vi "XYStage.KIM101.GetProtectedEvents.vi"(8 "error in (no error)":errorcluster, 11 "XYStage.KIM101":refnum<class "XYStage.KIM101.lvclass">) -> (0 "error out":errorcluster, 2 "Protected Events":T1, 3 "XYStage.KIM101 out":refnum<class "XYStage.KIM101.lvclass">)   [LabVIEW 2017, in "XYStage.KIM101.lvclass"]
doc: "---------------------------------------------------------------\nJKI State Machine Objects™\nhttp://jki.net/state-machine-objects/\nCopyright (C) 2005-2015, JKI <info@jki.net>\nALL RIGHTS RESERVEDJKI State Machine Objects (SMO) 1.0.0.5\nJKI - JKI\nCopyright (c) 2016, JKI"
uses:
  XYStage.KIM101.lvclass
  Typedefs/ProtectedEvents--Cluster.ctl
  Typedefs/NewValueEvent--Cluster.ctl
  XYStage.KIM101.lvclass/XYStage.KIM101.ctl
panel:
  # "For instructions on how to use the JKI State Machine Objects, examples and video tutorials, visit:\nhttp://jki.net/state-machine-objects/\n\nJKI State Machine Objects™\nhttp://jki.net/state-machine-objects/\nCopyright (C) 2005-2015, JKI <info@jki.net>\nALL RIGHTS RESERVED"
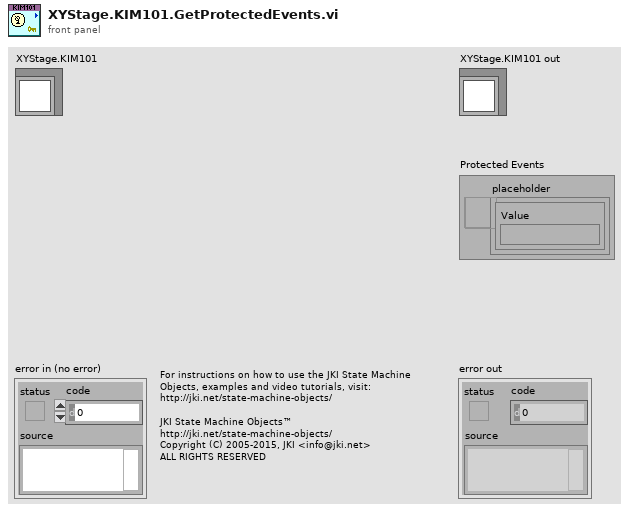
[diagram p1: front panel]
types:
  T1 = typedef "XYStage.KIM101.lvclass/ProtectedEvents--Cluster.ctl" = cluster{"placeholder":refnum<user-event>}
  T2 = typedef "XYStage.KIM101.lvclass/PrivateData--Ref.ctl" = refnum<data-value>
  T3 = typedef "XYStage.KIM101.lvclass/PrivateData--Cluster.ctl" = cluster{"Public Events":T4, "Protected Events":T1, "Private Events":T5, "Value":T6}
  T4 = typedef "XYStage.KIM101.lvclass/PublicEvents--Cluster.ctl" = cluster{"Value Changed":refnum<user-event>}
  T5 = typedef "XYStage.KIM101.lvclass/PrivateEvents--Cluster.ctl" = cluster{"New Value":refnum<user-event>}
  T6 = typedef "XYStage.KIM101.lvclass/Value.ctl" = string
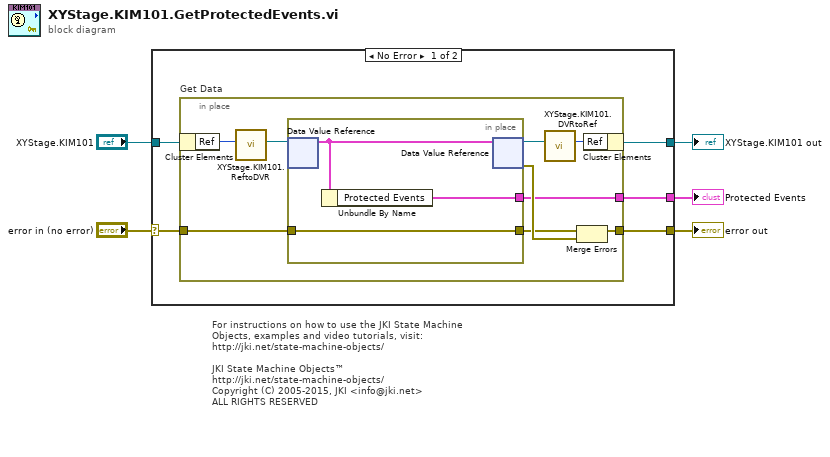
[diagram p0: block diagram]
diagram:
  # "For instructions on how to use the JKI State Machine Objects, examples and video tutorials, visit:\nhttp://jki.net/state-machine-objects/\n\nJKI State Machine Objects™\nhttp://jki.net/state-machine-objects/\nCopyright (C) 2005-2015, JKI <info@jki.net>\nALL RIGHTS RESERVED"
  n1 = case shown="No Error" "error in (no error)" {
    selector: "error in (no error)" -> [w9 w23]
    tunnel: "XYStage.KIM101" -> [w10 w24]
    tunnel: [w8 w23] -> w4
    tunnel: [w7 w24] -> w3
    tunnel: [w6 _] -> w1
    frame No Error {
      n2 = in-place "Get Data" {
        in-place-border: w9 -> [w19]
        in-place-border: [w16] -> w8
        in-place-border: [w15] -> w6
        n3 = in-place-cluster #1(w10) -> ("Ref"=w12:u32)
        n4 = call "XYStage.KIM101.ReftoDVR.vi"("Ref"=w12) -> ("Ref"=w11:T2)  [unwired: 10 in]
        n5 = in-place {
          in-place-border: w19 -> [w21]
          in-place-border: [w21] -> w17
          in-place-border: [w20] -> w15
          n6 = in-place-dvr #2(w11) -> (w22:T3)  [unwired: 1 out]
          n7 = Unbundle By Name(w22) -> ("Protected Events"=w20:T1)
          n8 = in-place-dvr #2(w22) -> (w14:T2, w18:errorcluster)
        }
        n9 = call "XYStage.KIM101.DVRtoRef.vi"("Ref"=w14) -> ("Ref"=w13:u32)  [unwired: 10 in]
        n10 = Merge Errors(w17, w18) -> (w16:errorcluster)
        n11 = in-place-cluster #1("Ref"=w13) -> (w7:refnum<class "XYStage.KIM101.lvclass">)
      }
    }
    frame Error {
    }
  }
  "error out" <- w4
  "XYStage.KIM101 out" <- w3
  "Protected Events" <- w1
